vi "SampleRate_Convert_GCFS.vi"(3 "Sample Rate":i32) -> (0 "Sample dt (s)":dbl, 1 "Sample dt (ms)":i64)   [LabVIEW 2024]
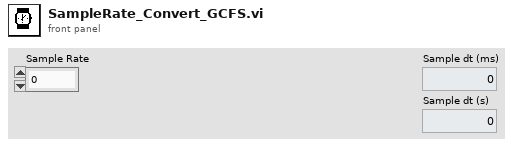
[diagram p1: front panel]
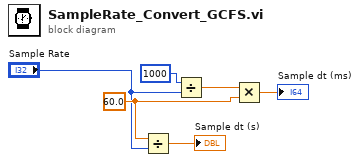
[diagram p0: block diagram]
diagram:
  w3 = 60.0 ("y")
  n1 = Divide(x=w3, y="Sample Rate") -> (x/y=→"Sample dt (s)":dbl)
  n2 = Divide(x=1000, y="Sample Rate") -> (x/y=w5:dbl)
  n3 = Multiply(x=w5, y=w3) -> (x*y=→"Sample dt (ms)":dbl)
